vi "MVP02 RT Driver VI.vi"(6 "Device Clock":string, 9 "Device Inputs FIFO":refnum<k33>, 10 "Device Outputs FIFO":refnum<k33>, 11 "Device Reference":T1 format="%.0x") -> ()   [LabVIEW 2016, in "MVP02 Custom Device.lvlib"]
uses:
  MVP02 Custom Device.lvlib
  <vilib>/NI Veristand/Custom Device API/Custom Device Item Ref.ctl
  <vilib>/NI Veristand/Custom Device API/Custom Device Channel Type.ctl
  <vilib>/NI Veristand/Custom Device API/Message Response (String).ctl
  <vilib>/NI Veristand/Custom Device API/Message Response (Byte Array).ctl
  <vilib>/NI Veristand/Custom Device API/Custom Device API.lvlib
  <vilib>/NI Veristand/Custom Device Tools/Custom Device Utility Library/Custom Device Utility Library.lvlib
panel:
  in  "Initialization Status Notifier":refnum<notifier>
  in  "Status Notifier":refnum<notifier>
  # "Custom Device Template\nv1.0"
  # "Use this template as a starting point for creating a custom device code module. The input controls shown here are specially named controls that the system will use to provide the device loop with data. The controls are not required for the device loop to run. For instance, if the device doesn't produce any output data, then you don't need the Device Outputs FIFO control. If you do use these controls, however, they need to have these exact names to be functional."
  # "The optional status notifier element is used to notify the RT engine of the last state of the custom device, and to indicate the device has completed execution. If this control is not used, a default No Error value is returned to the system when the device finishes execution.\n\nNote: This error state is not checked until the system shuts down. Use an output status channel to send more immediate status values to the system."
  # "This optional input can be used to send the VeriStand Engine the final status of the custom device initalization process. If this control exists on the custom device front panel, the VeriStand Engine will wait for a status update before starting up. If the custom device reports an error, that will abort the execution of the current configuration in the VeriStand Engine.\n\nThis control can be deleted if the custom device does not need to send the initialization status update."
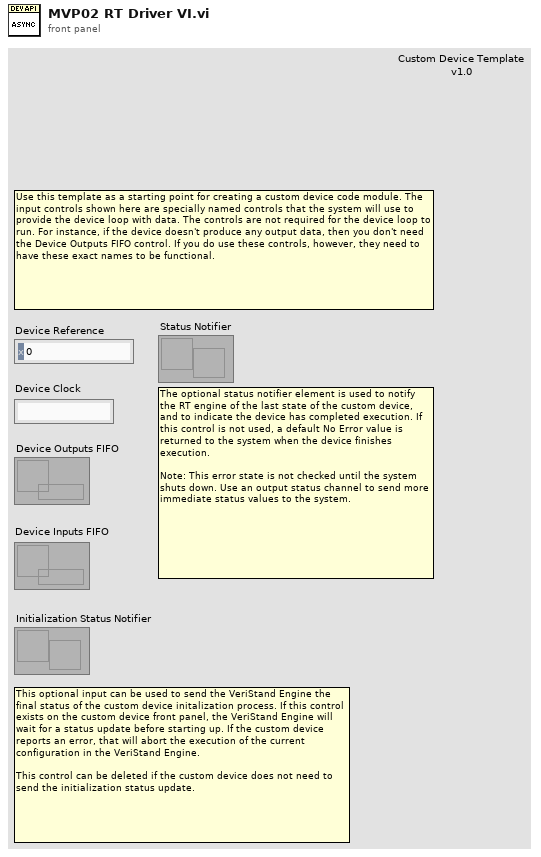
[diagram p1: front panel]
types:
  T1 = typedef "Custom Device API.lvlib/Custom Device Item Ref.ctl" = u64
  T2 = typedef "Custom Device API.lvlib/Custom Device Channel Type.ctl" = enum16{"Input", "Output"}
  T3 = typedef "Custom Device API.lvlib/Custom Device Engine Event Ref.ctl" = refnum<event-registration>
  T4 = enum16{"open", "open or create", "create or replace", "create", "open (read-only)"}
  T5 = enum16{"Sine Wave", "Triangle Wave", "Square Wave", "Sawtooth Wave"}
  T6 = typedef "Custom Device API.lvlib/Message Response (String).ctl" = cluster{"Response":string, "Error":errorcluster}
  T7 = typedef "Custom Device API.lvlib/Message Response (Byte Array).ctl" = cluster{"Response":u8[], "Error":errorcluster}
  T8 = typedef "Vision Case.ctl" = enum16{"Espera", "OCR", "OCR2", "Outros"}
  T9 = typedef "IMAQ Image.ctl" = refnum<image>
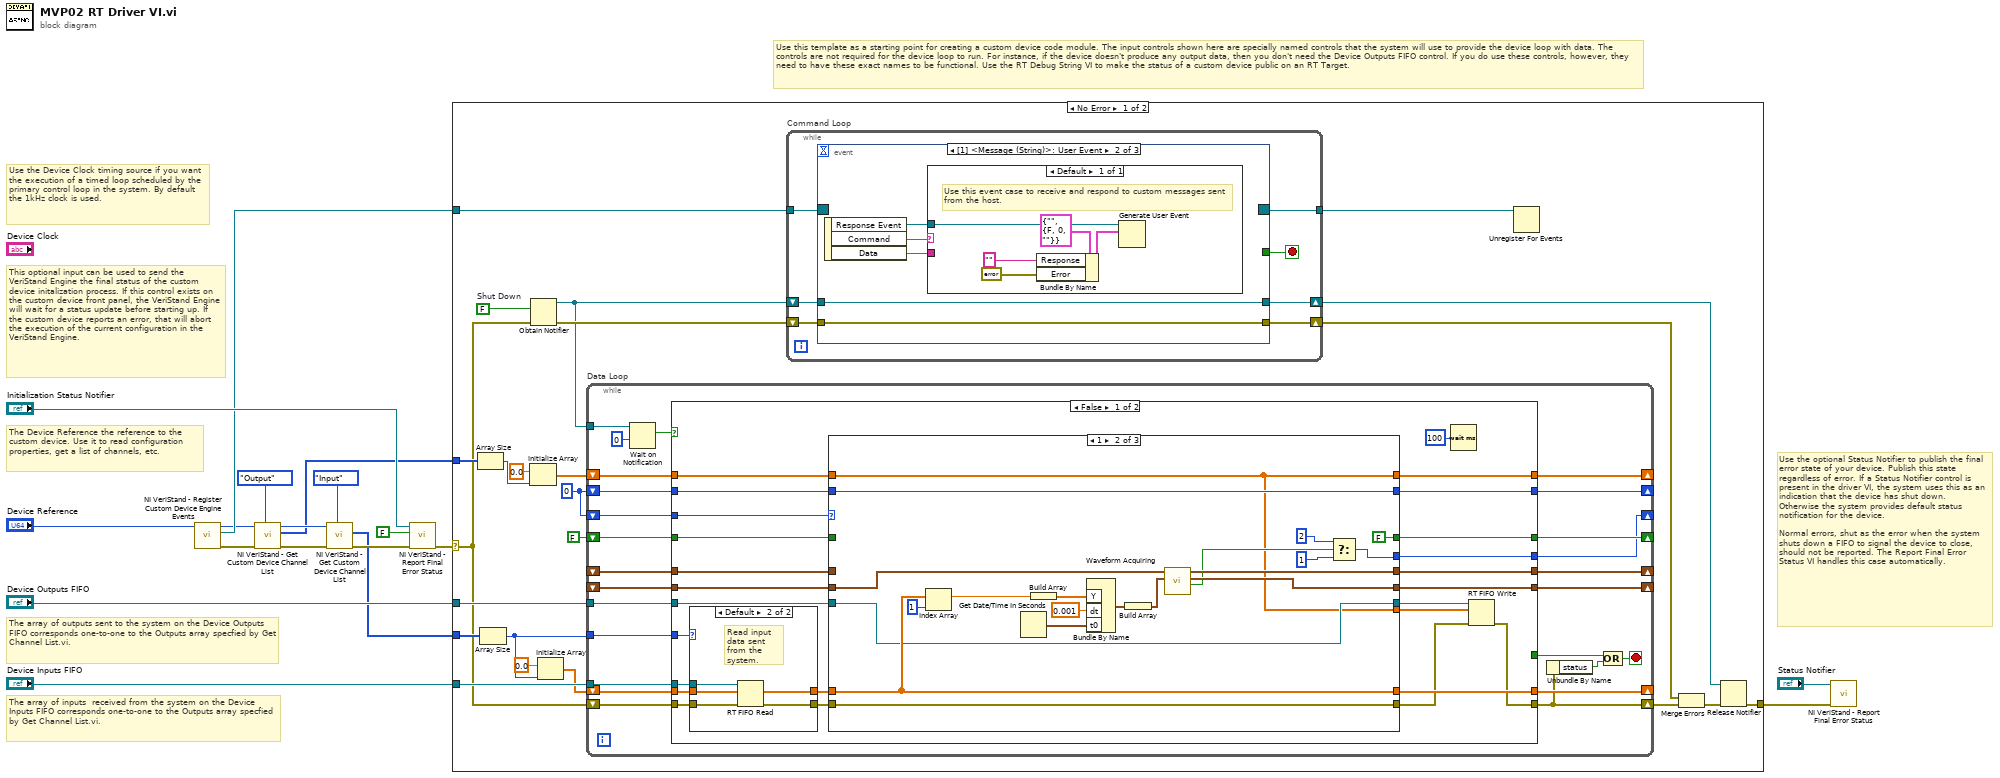
[diagram p0: block diagram]
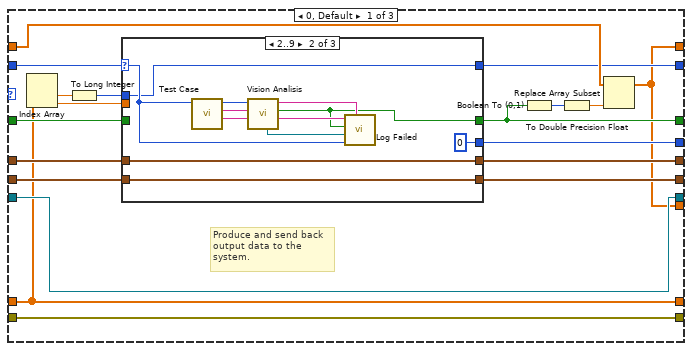
[diagram p2: hidden frame]
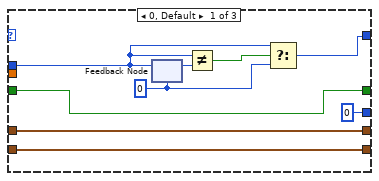
[diagram p3: hidden frame]
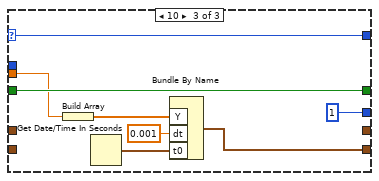
[diagram p4: hidden frame]
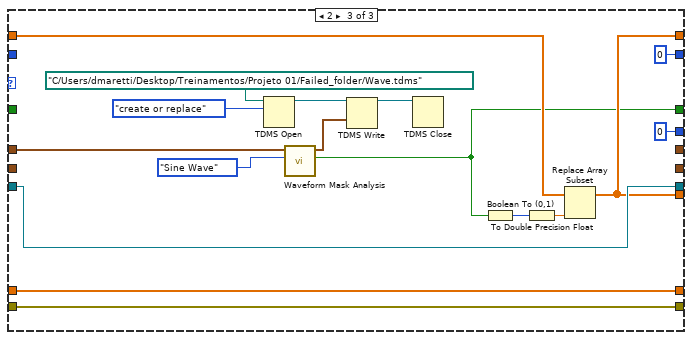
[diagram p5: hidden frame]
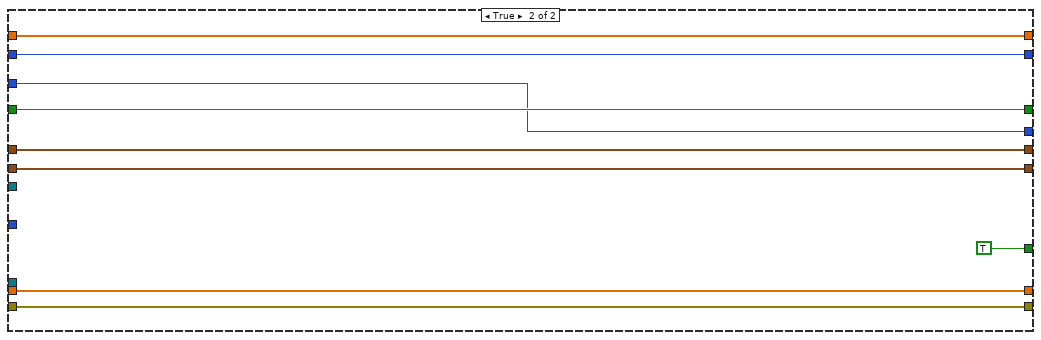
[diagram p7: hidden frame]
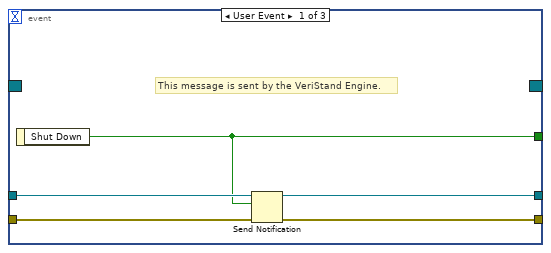
[diagram p8: hidden frame]
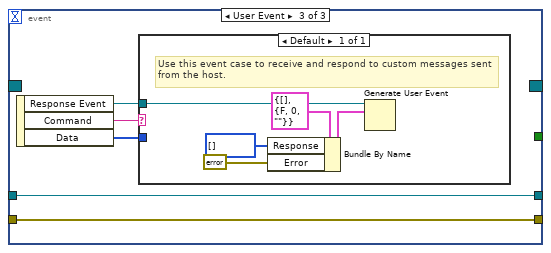
[diagram p9: hidden frame]
diagram:
  # "This optional input can be used to send the VeriStand Engine the final status of the custom device initalization process. If this control exists on the custom device front panel, the VeriStand Engine will wait for a status update before starting up. If the custom device reports an error, that will abort the execution of the current configuration in the VeriStand Engine."
  # "The array of inputs  received from the system on the Device Inputs FIFO corresponds one-to-one to the Outputs array specfied by Get Channel List.vi."
  # "Use the optional Status Notifier to publish the final error state of your device. Publish this state regardless of error. If a Status Notifier control is present in the driver VI, the system uses this as an indication that the device has shut down. Otherwise the system provides default status notification for the device.\n\nNormal errors, shut as the error when the system shuts down a FIFO to signal the device to close, should not be reported. The Report Final Error Status VI handles this case automatically."
  # "The array of outputs sent to the system on the Device Outputs FIFO corresponds one-to-one to the Outputs array specfied by Get Channel List.vi."
  # "The Device Reference the reference to the custom device. Use it to read configuration properties, get a list of channels, etc."
  # "Use the Device Clock timing source if you want the execution of a timed loop scheduled by the primary control loop in the system. By default the 1kHz clock is used."
  # "Use this template as a starting point for creating a custom device code module. The input controls shown here are specially named controls that the system will use to provide the device loop with data. The controls are not required for the device loop to run. For instance, if the device doesn't produce any output data, then you don't need the Device Outputs FIFO control. If you do use these controls, however, they need to have these exact names to be functional. Use the RT Debug String VI to make the status of a custom device public on an RT Target."
  n1 = call <vilib>:"NI VeriStand - Register Custom Device Engine Events.vi"("Device Ref in"="Device Reference") -> ("error out"=w18:errorcluster, "Custom Device Engine Event Ref"=w6:T3, "Device Ref out"=w3:T1)  [unwired: 8 in]
  n2 = call <vilib>:"NI VeriStand - Get Custom Device Channel List.vi"("Channel Type"=Custom_Device_Channel_Type."Output", "error in (no error)"=w18, "Device Ref in"=w3) -> ("error out"=w11:errorcluster, "Specified Channel Ref List"=w8:T1[], "Device Ref out"=w12:T1)  [unwired: 6 out]
  n3 = call <vilib>:"NI VeriStand - Get Custom Device Channel List.vi"("Channel Type"=Custom_Device_Channel_Type."Input", "error in (no error)"=w11, "Device Ref in"=w12) -> ("error out"=w17:errorcluster, "Specified Channel Ref List"=w9:T1[])  [unwired: 7 out]
  n4 = call <vilib>:"NI VeriStand - Report Final Error Status.vi"("error in (no error)"=w17, "Filter FIFO & Shutdown Errors (T)"=FALSE ("Filter FIFO Errors (T)"), "Status Notifier"="Initialization Status Notifier") -> ("error out"=w2:errorcluster)  [unwired: 8 out]
  n5 = case shown="No Error" w2 {
    selector: w2 -> [w20 w225]
    tunnel: "Device Outputs FIFO" -> [w40 _]
    tunnel: "Device Inputs FIFO" -> [w39 _]
    tunnel: w9 -> [w33 _]
    tunnel: w8 -> [w32 _]
    tunnel: w6 -> [w30 _]
    tunnel: [w28 w225] -> w5
    frame No Error {
      w19 = 0
      w29 = FALSE  # Shut Down
      n6 = Array Size(array=w32) -> (size(s)=w34:i32)
      n7 = Array Size(array=w33) -> (size(s)=w31:i32)
      n8 = Initialize Array(0.0 ("element"), w34) -> (w36:dbl[])
      n9 = Obtain Notifier(notification data type=w29, error in (no error)=w20) -> (notifier out=w26:refnum<notifier>, error out=w41:errorcluster)  [unwired: 2 in, 1 out]
      n10 = Initialize Array(0.0 ("element"), w31) -> (w35:dbl[])
      n11 = while "Data Loop" {
        shift-right: [w64] -> _
        shift-left: w35 -> [w65]
        shift-right: [w56] -> w24
        shift-left: w20 -> [w66]
        shift-right: [w62] -> _
        shift-left: w36 -> [w63]
        tunnel: w40 -> [w61]
        tunnel: w39 -> [w60]
        tunnel: w31 -> [w58]
        tunnel: w26 -> [w55]
        shift-right: [w50] -> _
        shift-left: FALSE ("Passed?") -> [w49]
        shift-right: [w48] -> _
        shift-left: _ -> [w47]
        shift-right: [w44] -> _
        shift-left: w19 -> [w59]
        shift-right: [w46] -> _
        shift-left: _ -> [w45]
        shift-right: [w42] -> _
        shift-left: w19 -> [w43]
        stop <- w51 stop-if-true
        n12 = Wait on Notification(notifier=w55, timeout in ms (-1)=0) -> (notification=w54:bool)  [unwired: 2 in, 3 out]
        n13 = case shown="False" w54 {
          tunnel: w66 -> [w91 w191]
          tunnel: w65 -> [w90 w192]
          tunnel: [w89 w192] -> w64
          tunnel: w63 -> [w88 w190]
          tunnel: [w87 w190] -> w62
          tunnel: w61 -> [w86 _]
          tunnel: w60 -> [w85 _]
          tunnel: w59 -> [w69 w187]
          tunnel: w58 -> [w84 _]
          tunnel: [w72 w191] -> w56
          tunnel: [_ TRUE] -> w52
          tunnel: [w80 w188] -> w50
          tunnel: w49 -> [w70 w188]
          tunnel: [w79 w184] -> w48
          tunnel: w47 -> [w78 w184]
          tunnel: [w77 w185] -> w46
          tunnel: w45 -> [w76 w185]
          tunnel: [w71 w187] -> w44
          tunnel: w43 -> [w68 w186]
          tunnel: [w67 w186] -> w42
          frame False {
            n14 = case shown="Default" w84 {
              tunnel: w85 -> [_ w183]
              tunnel: w90 -> [w178 w182]
              tunnel: [w178 w181] -> w83
              tunnel: [w177 w180] -> w82
              tunnel: w91 -> [w177 w179]
              frame 0 {
                # "No inputs to read\nfrom system. Inputs FIFO not created in this case, so don't write to it."
              }
              frame Default {
                # "Read input data sent from the system."
                n15 = RT FIFO Read(0:w183, 1:w182, 3:w179) -> (9:w181:dbl[], 11:w180:errorcluster)  [unwired: 4 out]
              }
            }
            n16 = case shown="1" w68 {
              tunnel: w86 -> [w105 w147 w174]
              tunnel: w88 -> [w104 w140 w171]
              tunnel: w83 -> [w97 w148 w172]
              tunnel: w82 -> [w106 w149 w173]
              tunnel: [w106 w149 w173] -> w73
              tunnel: [w92 w140 w168] -> w87
              tunnel: [w97 w148 w172] -> w89
              tunnel: [w108 FALSE ("test passed?") w167] -> w80
              tunnel: [w107 w151 _] -> w79
              tunnel: w78 -> [w99 w152 _]
              tunnel: [w101 w150 _] -> w77
              tunnel: w76 -> [w100 _ w176]
              tunnel: [w105 w147 w174] -> w75
              tunnel: [w92 w140 w168] -> w74
              tunnel: w69 -> [w103 w146 _]
              tunnel: [w102 w146 0] -> w71
              tunnel: w70 -> [w98 _ _]
              tunnel: [w95 w143 0] -> w67
              frame 0, Default {
                # "Produce and send back output data to the system."
                n17 = Index Array(array=w97) -> (element #1=w94:dbl, element #2=w96:dbl)  [unwired: 2 in]
                n18 = To Long Integer(number=w94) -> (32bit integer=w93:i32)
                n19 = case shown="2..9" w103 {
                  selector: w103 -> [_ w125 w136]
                  tunnel: [w113 w124 w134] -> w108
                  tunnel: [w117 w122 w135] -> w107
                  tunnel: [w114 w120 w136] -> w102
                  tunnel: w98 -> [w113 _ w134]
                  tunnel: [w118 w123 _] -> w101
                  tunnel: w100 -> [w118 w123 _]
                  tunnel: w99 -> [w117 w122 _]
                  tunnel: w96 -> [_ _ w133]
                  tunnel: [0 0 1] -> w95
                  tunnel: w93 -> [w111 w120 _]
                  frame 0, Default {
                    w115 = 0
                    n20 = feedback #1(w115) -> (w119:i32)
                    n21 = feedback-in #1(w111) -> ()
                    n22 = Not Equal?(x=w111, y=w119) -> (x != y?=w116:bool)
                    n23 = Select(t=w111, s=w116, f=w115) -> (s? t:f=w114:i32)
                  }
                  frame 2..9 {
                    n24 = call "Test Case.vi"("Numeric"=w125) -> ("Linha 2"=w128:string, "Linha 1"=w127:string, "Image Case"=w126:T8)  [unwired: 8 in]
                    n25 = call "Vision Analisis.vi"("Linha 2"=w128, "Linha 1"=w127, "Image Case"=w126) -> ("Gabarito"=w131:string, "Passed?"=w124:bool, "String (OCR/OCV 1)"=w130:string, "Image Out"=w129:T9)  [unwired: 4 in, 1 out]
                    n26 = call "Log Failed.vi"("RESULTADO"=w130, "Case number"=w125, "Image In"=w129, "Boolean"=w124, "GABARITO"=w131) -> ()  [unwired: 7 in]
                  }
                  frame 10 {
                    n27 = Build Array(w133) -> (w139:dbl[])
                    n28 = Get Date/Time In Seconds() -> (seconds since 1Jan1904=w137:timestamp)
                    n29 = Bundle By Name("Y"=w139, "dt"=0.001, "t0"=w137) -> (w135:waveform(dbl))  [unwired: 1 in]
                  }
                }
                n30 = Boolean To (0,1)(Boolean=w108) -> (0, 1=w110:i16)
                n31 = To Double Precision Float(number=w110) -> (double precision float=w109:dbl)
                n32 = Replace Array Subset(array=w104, new element=w109) -> (w92:dbl[])  [unwired: 1 in]
              }
              frame 1 {
                n33 = Index Array(array=w148, index=1) -> (element=w154:dbl)
                n34 = Get Date/Time In Seconds() -> (seconds since 1Jan1904=w159:timestamp)
                n35 = Build Array(w154) -> (w155:dbl[])
                n36 = Bundle By Name("Y"=w155, "dt"=0.001, "t0"=w159) -> (w157:waveform(dbl))  [unwired: 1 in]
                n37 = Build Array(w157) -> (w156:waveform(dbl)[])
                n38 = call "Waveform Acquiring.vi"("data"=w156, "waveform out 3"=w152) -> ("Boolean"=w142:bool, "waveform out 2"=w151:waveform(dbl), "waveform out"=w150:waveform(dbl))  [unwired: 7 in]
                n39 = Select(t=2, s=w142, f=1) -> (s? t:f=w143:i32)
              }
              frame 2 {
                n40 = TDMS Open(10:T4."create or replace" ("operation (0:open)"), 11:path "C:/Users/dmaretti/Desktop/Treinamentos/Projeto 01/Failed_folder/Wave.tdms" ("file path")) -> (3:w166:refnum<k34>)  [unwired: 5 in, 1 out]
                n41 = call "Waveform Mask Analysis.vi"("signal type"=T5."Sine Wave", "waveform in"=w176) -> ("test passed?"=w167:bool, "output values"=w160:waveform(dbl)[])  [unwired: 8 in]
                n42 = TDMS Write(0:w166, 9:w160) -> (4:w165:refnum<k34>)  [unwired: 4 in, 3 out]
                n43 = TDMS Close(11:w165) -> ()  [unwired: 1 in, 2 out]
                n44 = Boolean To (0,1)(Boolean=w167) -> (0, 1=w161:i16)
                n45 = To Double Precision Float(number=w161) -> (double precision float=w175:dbl)
                n46 = Replace Array Subset(array=w171, new element=w175) -> (w168:dbl[])  [unwired: 1 in]
              }
            }
            n47 = Wait (ms)(milliseconds to wait=u32 100) -> ()  [unwired: 1 out]
            n48 = RT FIFO Write(0:w75, 1:w74, 3:w73) -> (11:w72:errorcluster)  [unwired: 1 in, 4 out]
          }
          frame True {
          }
        }
        n49 = Unbundle By Name(w56) -> ("status"=w53:bool)
        n50 = Compound Arithmetic op=OR(w52, w53) -> (w51:bool)
      }
      n51 = while "Command Loop" {
        tunnel: w30 -> [w199]
        tunnel: [w198] -> w27
        shift-right: [w195] -> w25
        shift-left: w26 -> [w196]
        shift-right: [w193] -> w22
        shift-left: w41 -> [w194]
        stop <- w197 stop-if-true
        n52 = event shown="[1] <Message (String)>: User Event" {
          selector: w199 -> [_ _ _]
          dyn-events: [_ _ _] -> w198
          timeout: _ -> [_ _ _]
          tunnel: [w202 _ _] -> w197
          tunnel: w196 -> [w203 w207 w217]
          tunnel: [w204 w207 w217] -> w195
          tunnel: w194 -> [w201 w205 w215]
          tunnel: [w200 w205 w215] -> w193
          event User Event {
            # "This message is sent by the VeriStand Engine."
            n53 = event-data() -> ("Shut Down"=w202:bool)  [unwired: 1 in]
            n54 = Send Notification(notification=w202, notifier=w203, error in (no error)=w201) -> (notifier out=w204:refnum<notifier>, error out=w200:errorcluster)
          }
          event User Event {
            n55 = event-data() -> ("Response Event"=w206:refnum<user-event>, "Command"=w209:string, "Data"=w208:string)  [unwired: 1 in]
            n56 = case shown="Default" w209 {
              tunnel: w208 -> [_]
              tunnel: w206 -> [w214]
              frame Default {
                # "Use this event case to receive and respond to custom messages sent from the host."
                n57 = Bundle By Name(cluster=T6 {"Response"="", "Error"={"status"=FALSE, "code"=0, "source"=""}} ("event data"), "Response"="", "Error"=errorcluster {"status"=FALSE, "code"=0, "source"=""}) -> (w212:T6)
                n58 = Generate User Event(user event=w214, event data cluster=w212) -> ()  [unwired: 2 in, 2 out]
              }
            }
          }
          event User Event {
            n59 = event-data() -> ("Response Event"=w216:refnum<user-event>, "Command"=w219:string, "Data"=w218:u8[])  [unwired: 1 in]
            n60 = case shown="Default" w219 {
              tunnel: w218 -> [_]
              tunnel: w216 -> [w224]
              frame Default {
                # "Use this event case to receive and respond to custom messages sent from the host."
                n61 = Bundle By Name(cluster=T7 {"Response"=[], "Error"={"status"=FALSE, "code"=0, "source"=""}} ("event data"), "Response"=u8[] [], "Error"=errorcluster {"status"=FALSE, "code"=0, "source"=""}) -> (w221:T7)
                n62 = Generate User Event(user event=w224, event data cluster=w221) -> ()  [unwired: 2 in, 2 out]
              }
            }
          }
        }
      }
      n63 = Unregister For Events(event registration refnum=w27) -> ()  [unwired: 1 in, 1 out]
      n64 = Merge Errors(w22, w24) -> (w23:errorcluster)
      n65 = Release Notifier(notifier=w25, error in (no error)=w23) -> (error out=w28:errorcluster)  [unwired: 1 in, 2 out]
    }
    frame Error {
    }
  }
  n66 = call <vilib>:"NI VeriStand - Report Final Error Status.vi"("error in (no error)"=w5, "Status Notifier"="Status Notifier") -> ()  [unwired: 1 in, 9 out]
